vi "Pick Found Method Names.vi"(2 "delimiter":string=":", 5 "Project Item Names":string[](array[string])=["Parrent.lvclass [My Computer< Untitled Project 1.lvproj]", "Child.lvclass [My Computer< Untitled Project 1.lvproj]", "QD Test.vi [My Computer< Untitled Project 1.lvproj]", "Find Project Items.vi [QuickDrop< My Computer< Untitled Project 1.lvproj]", "Get Default QD Object Shortcuts File.vi [QuickDrop< My Computer< Untitled Project 1.lvproj]", "Load Default QD Object Shortcuts.vi [QuickDrop< My Computer< Untitled Project 1.lvproj]", "OldSearchAlgorithm.vi [QuickDrop< My Computer< Untitled Project 1.lvproj]", "OpenSearchWrapper.vi [QuickDrop< My Computer< Untitled Project 1.lvproj]", "QuickDrop Get QDKS Info for Shortcut Dialog.vi [QuickDrop< My Computer< Untitled Project 1.lvproj]", "QuickDrop Get QDKS Mappings.vi [QuickDrop< My Computer< Untitled Project 1.lvproj]", "QuickDrop Get Shortcut Info.vi [QuickDrop< My Computer< Untitled Project 1.lvproj]", "QuickDrop Get Terminal Names.vi [QuickDrop< My Computer< Untitled Project 1.lvproj]", "QuickDrop Get Wire Prefix.vi [QuickDrop< My Computer< Untitled Project 1.lvproj]", "QuickDrop Launch Window.vi [QuickDrop< My Computer< Untitled Project 1.lvproj]", "QuickDrop Get Wire Query terms.vi [QuickDrop< My Computer< Untitled Project 1.lvproj]", "QuickDrop Insert String into Array.vi [QuickDrop< My Computer< Untitled Project 1.lvproj]", "QuickDrop Plugin Template.vit [QuickDrop< My Computer< Untitled Project 1.lvproj]", "QuickDrop Populate QDKS Listbox.vi [QuickDrop< My Computer< Untitled Project 1.lvproj]", "QuickDrop Process Drop Information.vi [QuickDrop< My Computer< Untitled Project 1.lvproj]", "QuickDrop QDKS Info.ctl [QuickDrop< My Computer< Untitled Project 1.lvproj]", "QuickDrop Read QDKS INI Info.vi [QuickDrop< My Computer< Untitled Project 1.lvproj]", "QuickDrop Shortcut Config.vi [QuickDrop< My Computer< Untitled Project 1.lvproj]", "QuickDrop Get Wire Class Query terms.vi [QuickDrop< My Computer< Untitled Project 1.lvproj]", "Parrent_Create.vi [Parrent.lvclass< My Computer< Untitled Project 1.lvproj]", "Destroy.vi [Parrent.lvclass< My Computer< Untitled Project 1.lvproj]", "Child_Create.vi [Child.lvclass< My Computer< Untitled Project 1.lvproj]", "Destroy.vi [Child.lvclass< My Computer< Untitled Project 1.lvproj]", "Method 1.vi [Child.lvclass< My Computer< Untitled Project 1.lvproj]", "Method 2.vi [Child.lvclass< My Computer< Untitled Project 1.lvproj]", "LV Config Read.vi [Dependencies< My Computer< Untitled Project 1.lvproj]", "LV Config Read Boolean.vi [Dependencies< My Computer< Untitled Project 1.lvproj]", "LV Config Read String.vi [Dependencies< My Computer< Untitled Project 1.lvproj]", "LV Config Read Pathlist.vi [Dependencies< My Computer< Untitled Project 1.lvproj]", "LV Config Read Color.vi [Dependencies< My Computer< Untitled Project 1.lvproj]", "LV Config Read Numeric (I32).vi [Dependencies< My Computer< Untitled Project 1.lvproj]", "LV Config Write.vi [Dependencies< My Computer< Untitled Project 1.lvproj]", "LV Config Write Boolean.vi [Dependencies< My Computer< Untitled Project 1.lvproj]", "LV Config Write String.vi [Dependencies< My Computer< Untitled Project 1.lvproj]", "LV Config Write Pathlist.vi [Dependencies< My Computer< Untitled Project 1.lvproj]", "LV Config Write Color.vi [Dependencies< My Computer< Untitled Project 1.lvproj]", "LV Config Write Numeric (I32).vi [Dependencies< My Computer< Untitled Project 1.lvproj]", "VSI TSVN Tbar_SVN Lock with Dialog.vi [Dependencies< My Computer< Untitled Project 1.lvproj]", "VSI TSVN Tbar_Handle SVN Error.vi [Dependencies< My Computer< Untitled Project 1.lvproj]", "Status Dialog Display Button.vi [Dependencies< My Computer< Untitled Project 1.lvproj]", "Status Dialog Justify Text.vi [Dependencies< My Computer< Untitled Project 1.lvproj]", "Status Dialog Update Message.vi [Dependencies< My Computer< Untitled Project 1.lvproj]", "Status Dialog Exit.vi [Dependencies< My Computer< Untitled Project 1.lvproj]", "Status Dialog Init.vi [Dependencies< My Computer< Untitled Project 1.lvproj]", "Status Dialog Wait for Status Queue.vi [Dependencies< My Computer< Untitled Project 1.lvproj]", "Status Dialog.vi [Dependencies< My Computer< Untitled Project 1.lvproj]", "Insert.vi [plugins< QuickDrop< My Computer< Untitled Project 1.lvproj]", "Move Labels.vi [plugins< QuickDrop< My Computer< Untitled Project 1.lvproj]", "Remove and Rewire.vi [plugins< QuickDrop< My Computer< Untitled Project 1.lvproj]", "Replace.vi [plugins< QuickDrop< My Computer< Untitled Project 1.lvproj]", "SVN Commit.vi [plugins< QuickDrop< My Computer< Untitled Project 1.lvproj]", "SVN Lock.vi [plugins< QuickDrop< My Computer< Untitled Project 1.lvproj]", "SVN Update.vi [plugins< QuickDrop< My Computer< Untitled Project 1.lvproj]", "VI Server Rename.vi [plugins< QuickDrop< My Computer< Untitled Project 1.lvproj]", "Wire All Terminals.vi [plugins< QuickDrop< My Computer< Untitled Project 1.lvproj]", "Wire Multiple Objects Together.vi [plugins< QuickDrop< My Computer< Untitled Project 1.lvproj]", "ObjectAttributes.ctl [protected< Parrent.lvclass< My Computer< Untitled Project 1.lvproj]", "Parrent_New.vi [utils< Parrent.lvclass< My Computer< Untitled Project 1.lvproj]", "Parrent_GetAttributes.vi [utils< Parrent.lvclass< My Computer< Untitled Project 1.lvproj]", "ObjectAttributes.ctl [protected< Child.lvclass< My Computer< Untitled Project 1.lvproj]", "Child_New.vi [utils< Child.lvclass< My Computer< Untitled Project 1.lvproj]", "Child_GetAttributes.vi [utils< Child.lvclass< My Computer< Untitled Project 1.lvproj]", "TTK_FTW-ERR-CallChain.vi [TTK_FTW.lvlib< Dependencies< My Computer< Untitled Project 1.lvproj]", "TTK_FTW-ERR-Clear.vi [TTK_FTW.lvlib< Dependencies< My Computer< Untitled Project 1.lvproj]", "TTK_FTW-ERR-NoErrorConstant.vi [TTK_FTW.lvlib< Dependencies< My Computer< Untitled Project 1.lvproj]", "TTK_FTW-ERR-ThrowError.vi [TTK_FTW.lvlib< Dependencies< My Computer< Untitled Project 1.lvproj]", "TTK_FTW-Regex-ReplaceAll.vi [TTK_FTW.lvlib< Dependencies< My Computer< Untitled Project 1.lvproj]", "TTK_FTW-Regex.vi [TTK_FTW.lvlib< Dependencies< My Computer< Untitled Project 1.lvproj]", "TTK_FTW-STR-Array-Delimit.vi [TTK_FTW.lvlib< Dependencies< My Computer< Untitled Project 1.lvproj]", "TTK_FTW-STR-ReplaceWhitespace.vi [TTK_FTW.lvlib< Dependencies< My Computer< Untitled Project 1.lvproj]", "Available Non-Node.ctl [_WireMultipleSupport< plugins< QuickDrop< My Computer< Untitled Project 1.lvproj]", "Change Tunnel Modes to Fix Wires.vi [_WireMultipleSupport< plugins< QuickDrop< My Computer< Untitled Project 1.lvproj]", "Connect Valid Terminals.vi [_WireMultipleSupport< plugins< QuickDrop< My Computer< Untitled Project 1.lvproj]", "Connector Pane Position.ctl [_WireMultipleSupport< plugins< QuickDrop< My Computer< Untitled Project 1.lvproj]", "Find Top and Error Terminals.vi [_WireMultipleSupport< plugins< QuickDrop< My Computer< Untitled Project 1.lvproj]", "Get Wirable Objects from Selection.vi [_WireMultipleSupport< plugins< QuickDrop< My Computer< Untitled Project 1.lvproj]", "Group Selection List By Row.vi [_WireMultipleSupport< plugins< QuickDrop< My Computer< Untitled Project 1.lvproj]", "Match Relaxed Data Type.vi [_WireMultipleSupport< plugins< QuickDrop< My Computer< Untitled Project 1.lvproj]", "Match Source and Sink Terminals.vi [_WireMultipleSupport< plugins< QuickDrop< My Computer< Untitled Project 1.lvproj]", "Node Terminal Info.ctl [_WireMultipleSupport< plugins< QuickDrop< My Computer< Untitled Project 1.lvproj]", "Node-Terminal Pair.ctl [_WireMultipleSupport< plugins< QuickDrop< My Computer< Untitled Project 1.lvproj]", "Prepare to Wire Two Nodes.vi [_WireMultipleSupport< plugins< QuickDrop< My Computer< Untitled Project 1.lvproj]", "Sort Node Terminals.vi [_WireMultipleSupport< plugins< QuickDrop< My Computer< Untitled Project 1.lvproj]", "Sort Unwired Terminals.vi [_WireMultipleSupport< plugins< QuickDrop< My Computer< Untitled Project 1.lvproj]", "What to Wire.ctl [_WireMultipleSupport< plugins< QuickDrop< My Computer< Untitled Project 1.lvproj]", "Wire Non-Nodes to Nodes.vi [_WireMultipleSupport< plugins< QuickDrop< My Computer< Untitled Project 1.lvproj]"], 9 "Method File Names":string[](array[string])) -> (8 "Method File Names":string[](array[string]))   [LabVIEW 2018]
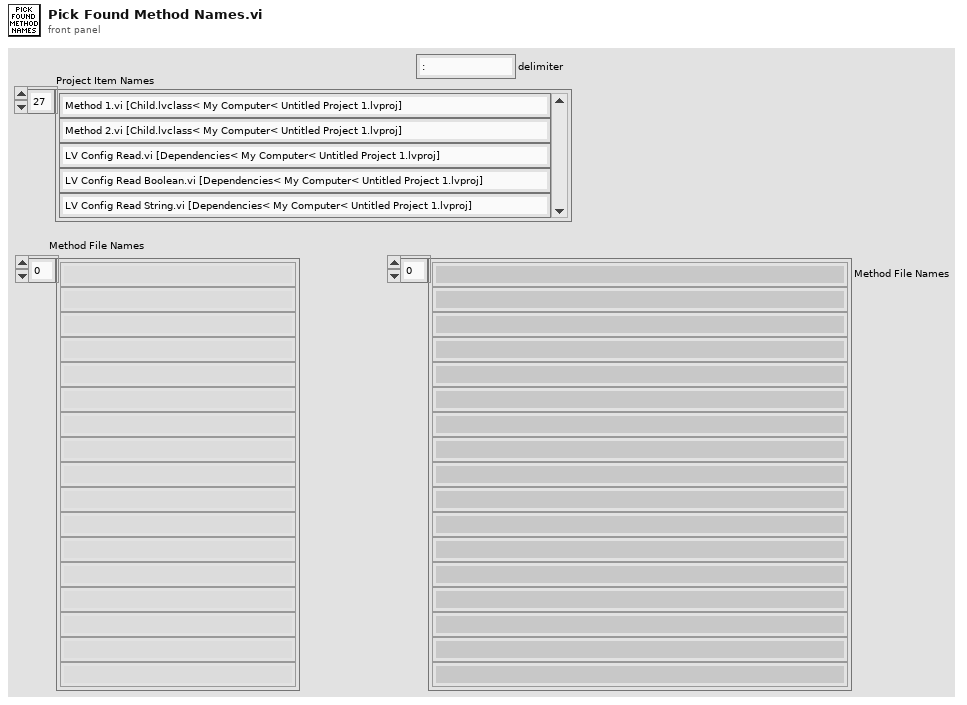
[diagram p1: front panel]
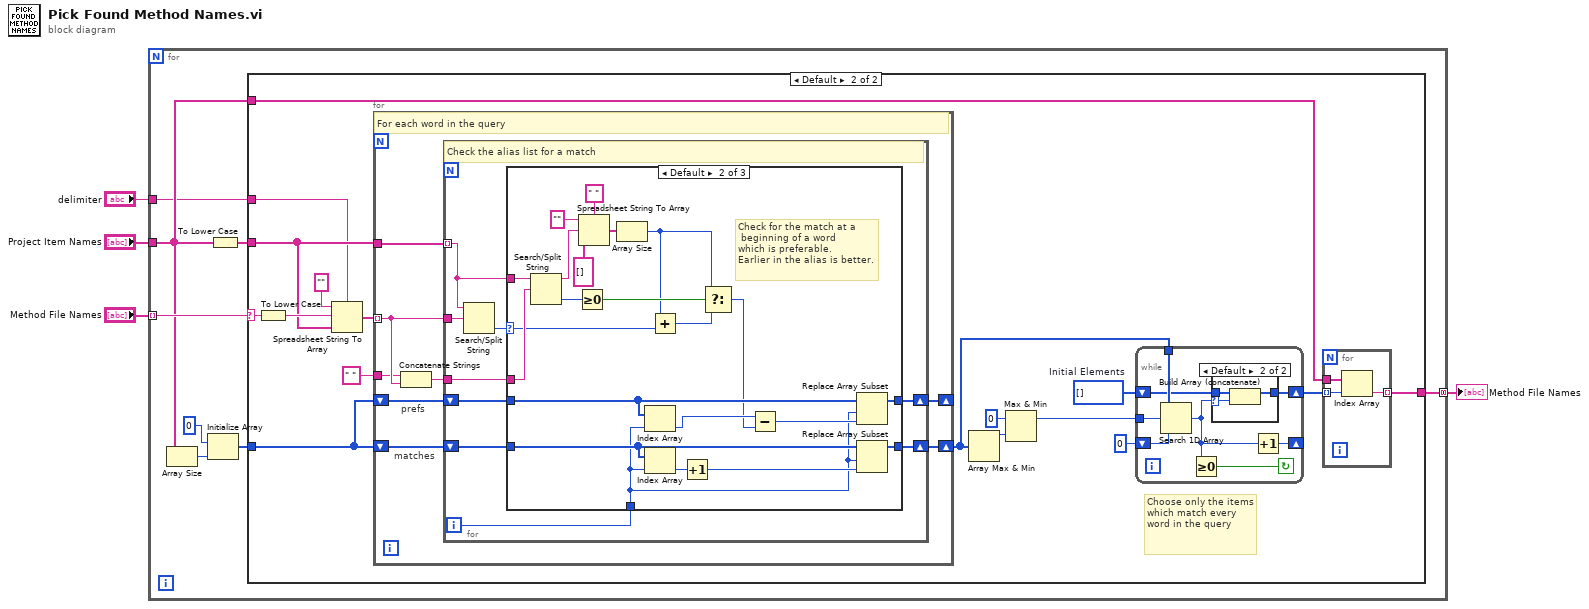
[diagram p0: block diagram]
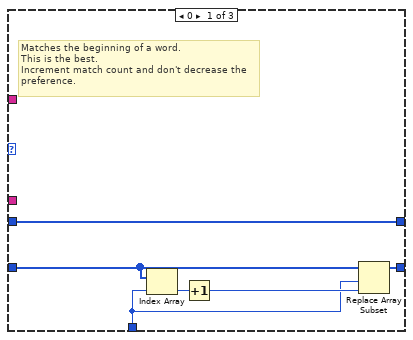
[diagram p4: hidden frame]
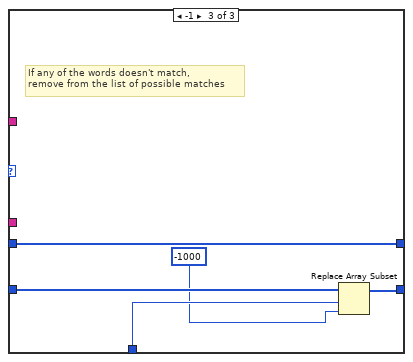
[diagram p5: hidden frame]
diagram:
  n1 = for {
    tunnel: "Project Item Names" -> [w7]
    tunnel: "Method File Names" -> [w8] mode=indexing
    tunnel: [w6] -> w2 mode=concatenating
    tunnel: "delimiter" -> [w5]
    n2 = Array Size(array=w7) -> (size(s)=w11:i32)
    n3 = Initialize Array(0, w11) -> (w9:i32[])
    n4 = To Lower Case(string=w7) -> (all lower case string=w12:string[])
    n5 = case shown="Default" w8 {
      selector: w8 -> [_ w23]
      tunnel: w7 -> [w13 w27]
      tunnel: [w13 w20] -> w6
      tunnel: w12 -> [_ w26]
      tunnel: w9 -> [_ w25]
      tunnel: w5 -> [_ w14]
      frame "" {
      }
      frame Default {
        w16 = i32[] []  # Initial Elements
        # "Choose only the items which match every word in the query"
        n6 = To Lower Case(string=w23) -> (all lower case string=w29:string)
        n7 = Spreadsheet String To Array(delimiter (Tab)=w14, format string="", spreadsheet string=w29, array type (2D Dbl)=w26) -> (array=w28:string[])
        n8 = for {
          tunnel: w26 -> [w53]
          tunnel: w28 -> [w48] mode=indexing
          shift-right: [w51] -> w17
          shift-left: w25 -> [w52]
          shift-right: [w49] -> _
          shift-left: w25 -> [w50]
          tunnel: " " ("delimiter (Tab)") -> [w47]
          # "matches"
          # "prefs"
          # "For each word in the query"
          n9 = Concatenate Strings(w47, w48) -> (w46:string)
          n10 = for {
            tunnel: w53 -> [w56] mode=indexing
            tunnel: w48 -> [w62]
            shift-right: [w59] -> w51
            shift-left: w52 -> [w60]
            shift-right: [w58] -> w49
            shift-left: w50 -> [w57]
            tunnel: w46 -> [w55]
            i -> [w61]
            # "Check the alias list for a match"
            n11 = Search/Split String(string=w56, search string/char (-)=w62) -> (offset of match=w54:i32)  [unwired: 1 in, 2 out]
            n12 = case shown="Default" w54 {
              selector: w54 -> [_ w72 _]
              tunnel: w61 -> [w64 w73 w93]
              tunnel: w60 -> [w67 w89 w94]
              tunnel: [w68 w90 w91] -> w59
              tunnel: [w63 w85 w95] -> w58
              tunnel: w57 -> [w63 w86 w95]
              tunnel: w56 -> [_ w82 _]
              tunnel: w55 -> [_ w81 _]
              frame 0 {
                # "Matches the beginning of a word. \nThis is the best.\nIncrement match count and don't decrease the preference."
                n13 = Index Array(array=w67, index=w64) -> (element=w66:i32)
                n14 = Increment(x=w66) -> (x+1=w65:i32)
                n15 = Replace Array Subset(array=w67, new element=w65, index=w64) -> (w68:i32[])
              }
              frame Default {
                # "Check for the match at a\n beginning of a word \nwhich is preferable.\nEarlier in the alias is better."
                n16 = Search/Split String(string=w82, search string/char (-)=w81) -> (substring before match=w75:string, offset of match=w80:i32)  [unwired: 1 in, 1 out]
                n17 = Greater Or Equal To 0?(x=w80) -> (x >= 0?=w79:bool)
                n18 = Spreadsheet String To Array(delimiter (Tab)=" ", format string="", spreadsheet string=w75, array type (2D Dbl)=string[] [] ("array")) -> (array=w74:string[])
                n19 = Array Size(array=w74) -> (size(s)=w69:i32)
                n20 = Index Array(array=w86, index=w73) -> (element=w84:i32)
                n21 = Index Array(array=w89, index=w73) -> (element=w88:i32)
                n22 = Add(x=w69, y=w72) -> (x+y=w70:i32)
                n23 = Increment(x=w88) -> (x+1=w87:i32)
                n24 = Select(t=w69, s=w79, f=w70) -> (s? t:f=w78:i32)
                n25 = Subtract(x=w84, y=w78) -> (x-y=w83:i32)
                n26 = Replace Array Subset(array=w86, new element=w83, index=w73) -> (w85:i32[])
                n27 = Replace Array Subset(array=w89, new element=w87, index=w73) -> (w90:i32[])
              }
              frame -1 {
                # "If any of the words doesn't match, \nremove from the list of possible matches"
                n28 = Replace Array Subset(array=w94, new element=-1000 ("new element/subarray"), index=w93) -> (w91:i32[])
              }
            }
          }
        }
        n29 = Array Max & Min(array=w17) -> (max value=w22:i32)  [unwired: 3 out]
        n30 = Max & Min(x=0, y=w22) -> (max(x,y)=w18:i32)  [unwired: 1 out]
        n31 = while {
          shift-right: [w31] -> _
          shift-left: 0 -> [w38]
          shift-right: [w35] -> w19
          shift-left: w16 -> [w36]
          tunnel: w17 -> [w37]
          tunnel: w18 -> [w34]
          stop <- w32 continue-if-true
          n32 = Search 1D Array(1D array=w37, element=w34, start index (0)=w38) -> (index of element=w33:i32)
          n33 = Greater Or Equal To 0?(x=w33) -> (x >= 0?=w32:bool)
          n34 = case shown="Default" w33 {
            selector: w33 -> [_ w42]
            tunnel: w36 -> [w39 w41]
            tunnel: [w39 w40] -> w35
            frame -1 {
            }
            frame Default {
              n35 = Build Array (concatenate)(w41, w42) -> (w40:i32[])
            }
          }
          n36 = Increment(x=w33) -> (x+1=w31:i32)
        }
        n37 = for {
          tunnel: w19 -> [w43] mode=indexing
          tunnel: w27 -> [w45]
          tunnel: [w44] -> w20 mode=indexing
          n38 = Index Array(array=w45, index=w43) -> (element=w44:string)
        }
      }
    }
  }
  "Method File Names" <- w2
